vi "basic-exit-log.vi"(11 "Cluster":T1) -> ()   [LabVIEW 2015]
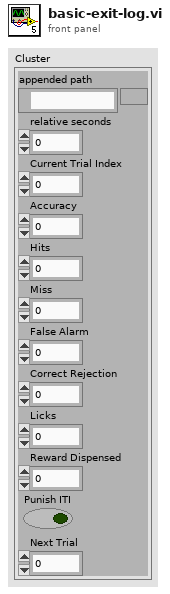
[diagram p1: front panel]
types:
  T1 = cluster{"appended path":path, "relative seconds":dbl, "Current Trial Index":i32, "Accuracy":dbl, "Hits":i32, "Miss":i32, "False Alarm":i32, "Correct Rejection":i32, "Licks":i32, "Reward Dispensed":dbl, "Punish ITI":bool, "Next Trial":i32}
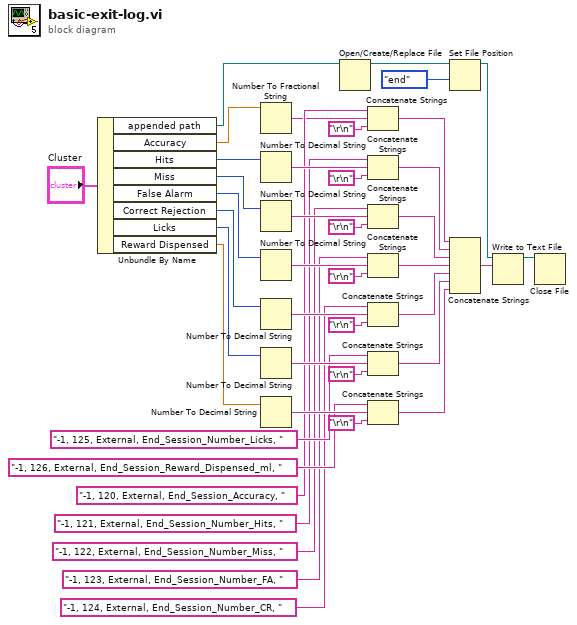
[diagram p0: block diagram]
diagram:
  n1 = Unbundle By Name("Cluster") -> ("appended path"=w41:path, "Accuracy"=w1:dbl, "Hits"=w2:i32, "Miss"=w3:i32, "False Alarm"=w4:i32, "Correct Rejection"=w5:i32, "Licks"=w6:i32, "Reward Dispensed"=w7:dbl)
  n2 = Number To Fractional String(number=w1) -> (F-format string=w8:string)  [unwired: 3 in]
  n3 = Number To Decimal String(number=w2) -> (decimal integer string=w11:string)  [unwired: 1 in]
  n4 = Number To Decimal String(number=w3) -> (decimal integer string=w13:string)  [unwired: 1 in]
  n5 = Number To Decimal String(number=w4) -> (decimal integer string=w15:string)  [unwired: 1 in]
  n6 = Number To Decimal String(number=w5) -> (decimal integer string=w17:string)  [unwired: 1 in]
  n7 = Number To Decimal String(number=w6) -> (decimal integer string=w19:string)  [unwired: 1 in]
  n8 = Number To Decimal String(number=w7) -> (decimal integer string=w21:string)  [unwired: 1 in]
  n9 = Open/Create/Replace File(file path (use dialog)=w41) -> (refnum out=w39:refnum<file>)  [unwired: 5 in, 2 out]
  n10 = Concatenate Strings("-1, 120, External, End_Session_Accuracy, " ("text"), w8, "\r\n") -> (w29:string)
  n11 = Concatenate Strings("-1, 121, External, End_Session_Number_Hits, " ("text"), w11, "\r\n") -> (w30:string)
  n12 = Concatenate Strings("-1, 122, External, End_Session_Number_Miss, " ("text"), w13, "\r\n") -> (w31:string)
  n13 = Concatenate Strings("-1, 123, External, End_Session_Number_FA, " ("text"), w15, "\r\n") -> (w32:string)
  n14 = Concatenate Strings("-1, 124, External, End_Session_Number_CR, " ("text"), w17, "\r\n") -> (w33:string)
  n15 = Concatenate Strings("-1, 125, External, End_Session_Number_Licks, " ("text"), w19, "\r\n") -> (w34:string)
  n16 = Concatenate Strings("-1, 126, External, End_Session_Reward_Dispensed_ml, " ("text"), w21, "\r\n") -> (w35:string)
  n17 = Set File Position(refnum=w39, from (0:start)=enum16{"start", "end", "current"}."end") -> (refnum out=w37:refnum<file>)  [unwired: 2 in, 1 out]
  n18 = Concatenate Strings(w29, w30, w31, w32, w33, w34, w35) -> (w42:string)
  n19 = Write to Text File(file (use dialog)=w37, text=w42) -> (refnum out=w40:refnum<file>)  [unwired: 2 in, 2 out]
  n20 = Close File(refnum=w40) -> ()  [unwired: 1 in, 2 out]
